vi "_USB_CAN_UnPackage_.vi"(0 "source":u8[](array[numeric])) -> (1 "length":i32, 2 "Type":enum16{"数据帧", "远程帧"}(ring), 3 "Format":enum16{"标准帧", "扩展帧"}(ring), 4 "TimeStamp":u32, 5 "data":u8[](array[numeric]), 6 "ID":u32)   [LabVIEW 2011]
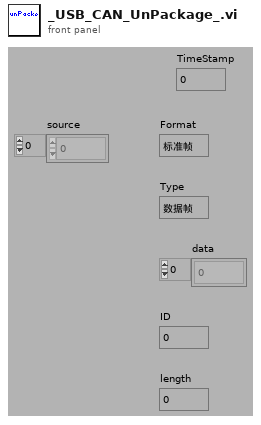
[diagram p1: front panel]
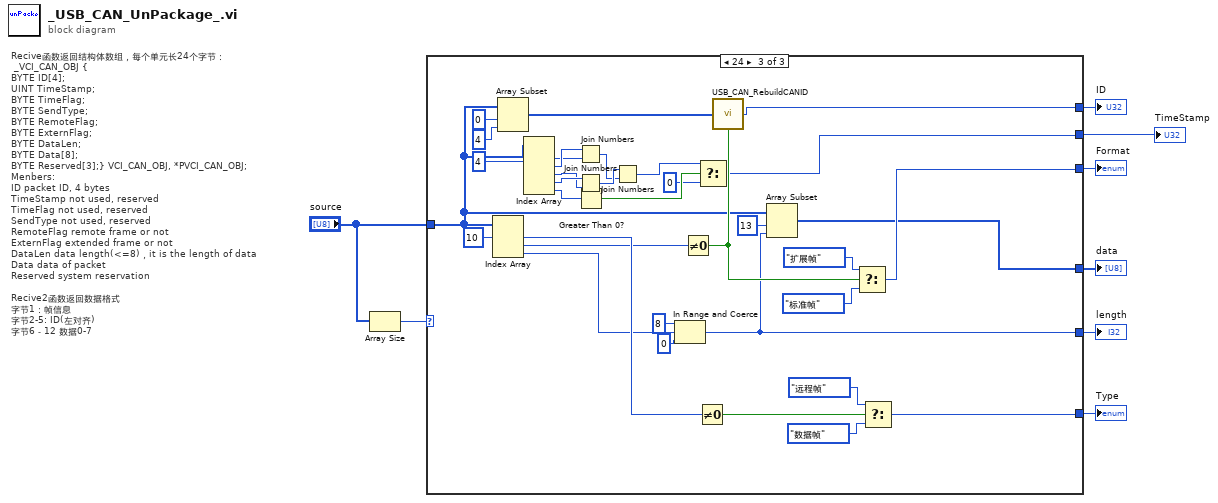
[diagram p0: block diagram]
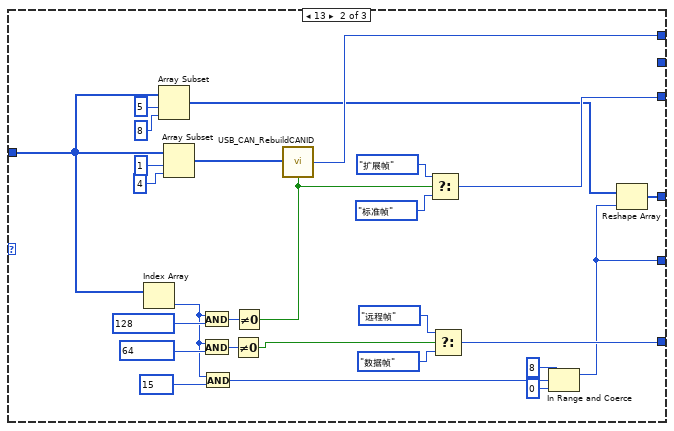
[diagram p3: hidden frame]
diagram:
  # "Recive函数返回结构体数组，每个单元长24个字节：\n _VCI_CAN_OBJ {\nBYTE ID[4];\nUINT TimeStamp;\nBYTE TimeFlag;\nBYTE SendType;\nBYTE RemoteFlag;\nBYTE ExternFlag;\nBYTE DataLen;\nBYTE Data[8];\nBYTE Reserved[3];} VCI_CAN_OBJ, *PVCI_CAN_OBJ;\nMenbers:\nID packet ID, 4 bytes\nTimeStamp not used, reserved\nTimeFlag not used, reserved\nSendType not used, reserved\nRemoteFlag remote frame or not\nExternFlag extended frame or not\nDataLen data length(<=8)，it is the length of data\nData data of packet\nReserved system reservation\n\nRecive2函数返回数据格式 \n字节1：帧信息\n字节2-5: ID(左对齐)\n字节6－12 数据0-7"
  n1 = Array Size(array="source") -> (size(s)=w3:i32)
  n2 = case shown="24" w3 {
    tunnel: [_ w35 w57] -> w8
    tunnel: "source" -> [_ w29 w48]
    tunnel: [_ w24 w56] -> w7
    tunnel: [_ w17 w62] -> w6
    tunnel: [_ w10 w53] -> w5
    tunnel: [_ w9 w50] -> w4
    tunnel: [_ _ w42] -> w1
    frame 0, Default {
    }
    frame 13 {
      n3 = Index Array(array=w29) -> (element=w16:u8)  [unwired: 1 in]
      n4 = Array Subset(array=w29, index=5, length=8) -> (w14:u8[])
      n5 = Array Subset(array=w29, index=1, length=4 ("长度")) -> (w30:u8[])
      n6 = And(x=w16, y=u8 128) -> (x .and. y?=w23:u8)
      n7 = And(x=w16, y=u8 64) -> (x .and. y?=w21:u8)
      n8 = And(x=w16, y=u8 15) -> (x .and. y?=w13:u8)
      n9 = Not Equal To 0?(x=w21) -> (x != 0?=w20:bool)
      n10 = Not Equal To 0?(x=w23) -> (x != 0?=w27:bool)
      n11 = call "USB_CAN_RebuildCANID.vi"("ExtFrame"=w27, "IDS"=w30) -> ("ID"=w35:u32)  [unwired: 2 in]
      n12 = Select(t=enum16{"标准帧", "扩展帧"}."扩展帧" ("Format"), s=w27, f=enum16{"标准帧", "扩展帧"}."标准帧" ("Format")) -> (s? t:f=w24:enum16{"标准帧", "扩展帧"})
      n13 = Select(t=enum16{"数据帧", "远程帧"}."远程帧" ("Type"), s=w20, f=enum16{"数据帧", "远程帧"}."数据帧" ("Type")) -> (s? t:f=w17:enum16{"数据帧", "远程帧"})
      n14 = In Range and Coerce(upper limit=u8 8 ("上限"), x=w13, lower limit=u8 0 ("下限")) -> (coerced(x)=w10:u8)  [unwired: 1 out]
      n15 = Reshape Array(w14, w10) -> (w9:u8[])
    }
    frame 24 {
      n16 = Index Array(array=w48, index #1=10 ("索引")) -> (element #1=w66:u8, element #2=w59:u8, element #3=w54:u8)  [unwired: 2 in]
      n17 = Array Subset(array=w48, index=0 ("索引"), length=4 ("长度")) -> (w49:u8[])
      n18 = Index Array(array=w48, index #1=4 ("索引")) -> (element #1=w40:u8, element #2=w41:u8, element #3=w38:u8, element #4=w39:u8, element #5=w46:u8)  [unwired: 4 in]
      n19 = Join Numbers(hi=w41, lo=w40) -> ((hi.lo)=w36:u16)
      n20 = Join Numbers(hi=w39, lo=w38) -> ((hi.lo)=w37:u16)
      n21 = Greater Than 0?(x=w46) -> (x > 0?=w45:bool)
      n22 = Join Numbers(hi=w37, lo=w36) -> ((hi.lo)=w44:u32)
      n23 = In Range and Coerce(upper limit=u8 8 ("上限"), x=w54, lower limit=u8 0 ("下限")) -> (coerced(x)=w53:u8)  [unwired: 1 out]
      n24 = Not Equal To 0?(x=w59) -> (x != 0?=w58:bool)
      n25 = Not Equal To 0?(x=w66) -> (x != 0?=w63:bool)
      n26 = Select(t=w44, s=w45, f=u32 0) -> (s? t:f=w42:u32)
      n27 = call "USB_CAN_RebuildCANID.vi"("ExtFrame"=w58, "IDS"=w49) -> ("ID"=w57:u32)  [unwired: 2 in]
      n28 = Array Subset(array=w48, index=13 ("索引"), length=w53) -> (w50:u8[])
      n29 = Select(t=enum16{"标准帧", "扩展帧"}."扩展帧" ("Format"), s=w58, f=enum16{"标准帧", "扩展帧"}."标准帧" ("Format")) -> (s? t:f=w56:enum16{"标准帧", "扩展帧"})
      n30 = Select(t=enum16{"数据帧", "远程帧"}."远程帧" ("Type"), s=w63, f=enum16{"数据帧", "远程帧"}."数据帧" ("Type")) -> (s? t:f=w62:enum16{"数据帧", "远程帧"})
    }
  }
  "Type" <- w6
  "Format" <- w7
  "ID" <- w8
  "length" <- w5
  "data" <- w4
  "TimeStamp" <- w1
